vi "FPGA Main.vi"() -> ()   [LabVIEW 2016]
doc: "This example transmits one frame contained in Data Frame every time the Write button is pressed. After building this FPGA VI, you run it using CAN Channel Transmit (Host).vi (not standalone).\n\nThis example assumes the following configuration for CAN 0: Auto Start = True, Listen Only = False, Input Timeout = 10000ms, Output Timeout = 10000ms. The CAN Output node is configured to use an array of U32 for the CAN frame. For more information on configuration, refer to the Help for the NI 9853 CAN module."
uses:
  <vilib>/rvi/eio/common/nirviEmuTemplateMethod_errors.vi
  <vilib>/rvi/Emulation/niFpgaCriticalErrorInLSC.vi
  <vilib>/rvi/eio/common/nirviEmuReportErrorAndStop.vi
  <vilib>/rvi/errors/nirviReportUnexpectedCaseInternalError.vi
  <vilib>/rvi/errors/nirviReportUnexpectedCaseInternalError (U32).vi
  <vilib>/rvi/Emulation/niFpgaProcessEmulError.vi
  <vilib>/rvi/occurrence/nirviWaitOnOccurrenceBase.vi
  <vilib>/rvi/FIFO/Fifo_Resource/nirvififoEmulationReleaseLock.vi
  <vilib>/rvi/FIFO/Fifo_Resource/nirvififoEmulationObtainLock.vi
  <vilib>/rvi/FIFO/Fifo_Resource/nirvififoEmulationCreateLock.vi
  <vilib>/rvi/DataTransferAndStorage/Container/Common/niFpgaContainerGetUniqueNameForEmu.vi
  <vilib>/rvi/FIFO/Fifo_Resource/nirvififoEmulationSetSize.vi
  <vilib>/Utility/error.llb/Clear Errors.vi
  <vilib>/rvi/FIFO/Fifo_Resource/nirviFifoEmulationQueueMgr.vi
  <instcachedir>/0/nirviFifoEmulationQueueMgr_E5CAEC123FF24DC58D834DCA3CDAA9B5.lvgen/nirviFifoEmulationQueueMgr_E5CAEC123FF24DC58D834DCA3CDAA9B5_009.vi
  <vilib>/rvi/errors/niFpgaSetErrorForExecOnDevCompSimple.vi
  <vilib>/rvi/Emulation/niFpgaSctlEmulationGetInTimedLoop.vi
  <vilib>/rvi/Emulation/niFpgaEmulationIsFPGAContextNoSignature.vi
  <vilib>/rvi/Emulation/niFpgaEmulationReportErrorSimple.vi
  <vilib>/rvi/Emulation/niFpgaGetClockAttributes.vi
  <vilib>/rvi/FIFO/Fifo_Resource/nirvififoEmulationDetermineInputValidOut.vi
  <vilib>/eio/EIONode/EIONode.xnode
  <vilib>/rvi/DataTransferAndStorage/Container/XNode/niFpgaContainer.xnode
  <vilib>/rvi/FIFO/Fifo_Resource/nirvififoEmulationRead.vi
  <vilib>/LabVIEW Targets/FPGA/RIO/nicrio_985x_controls.llb/CAN_IO_Frame Array U32.ctl
  <vilib>/rvi/FIFO/Fifo_Resource/nirvififoEmulationWrite.vi
  <vilib>/eio/EIOMethodNode/EIOMethodNode.xnode
  <vilib>/rvi/FIFO/Fifo_Resource/nirvififoEmulationClear.vi
panel:
  out "CAN Frame Out":T1 {"Data" format="%.0x"; "DataLength" format="%.0x"; "InfoB" format="%.0x"; "InfoA" format="%.0x"; "Type" format="%.0x"; "Identifier" format="%.0x"; "Timestamp" format="%.0x"}
  in  "CAN Frame In":T1={"Timestamp"=0, "Identifier"=0, "Type"=0, "InfoA"=0, "InfoB"=0, "DataLength"=0, "Data"=[0, 0, 0, 0, 0, 0, 0, 0]} {"Data" format="%.0x"; "DataLength" format="%.0x"; "InfoB" format="%.0x"; "InfoA" format="%.0x"; "Type" format="%.0x"; "Identifier" format="%.0x"; "Timestamp" format="%.0x"}
  out "FIFO Full":bool
  in  "Write":bool
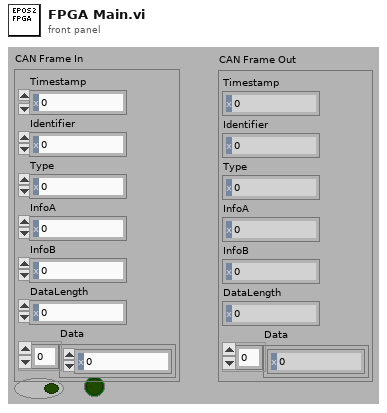
[diagram p1: front panel]
types:
  T1 = cluster{"Timestamp":u64, "Identifier":u32, "Type":u8, "InfoA":u8, "InfoB":u8, "DataLength":u8, "Data":u8[]}
  T2 = typedef "CAN_IO_Frame Array U32.ctl" = u32[]
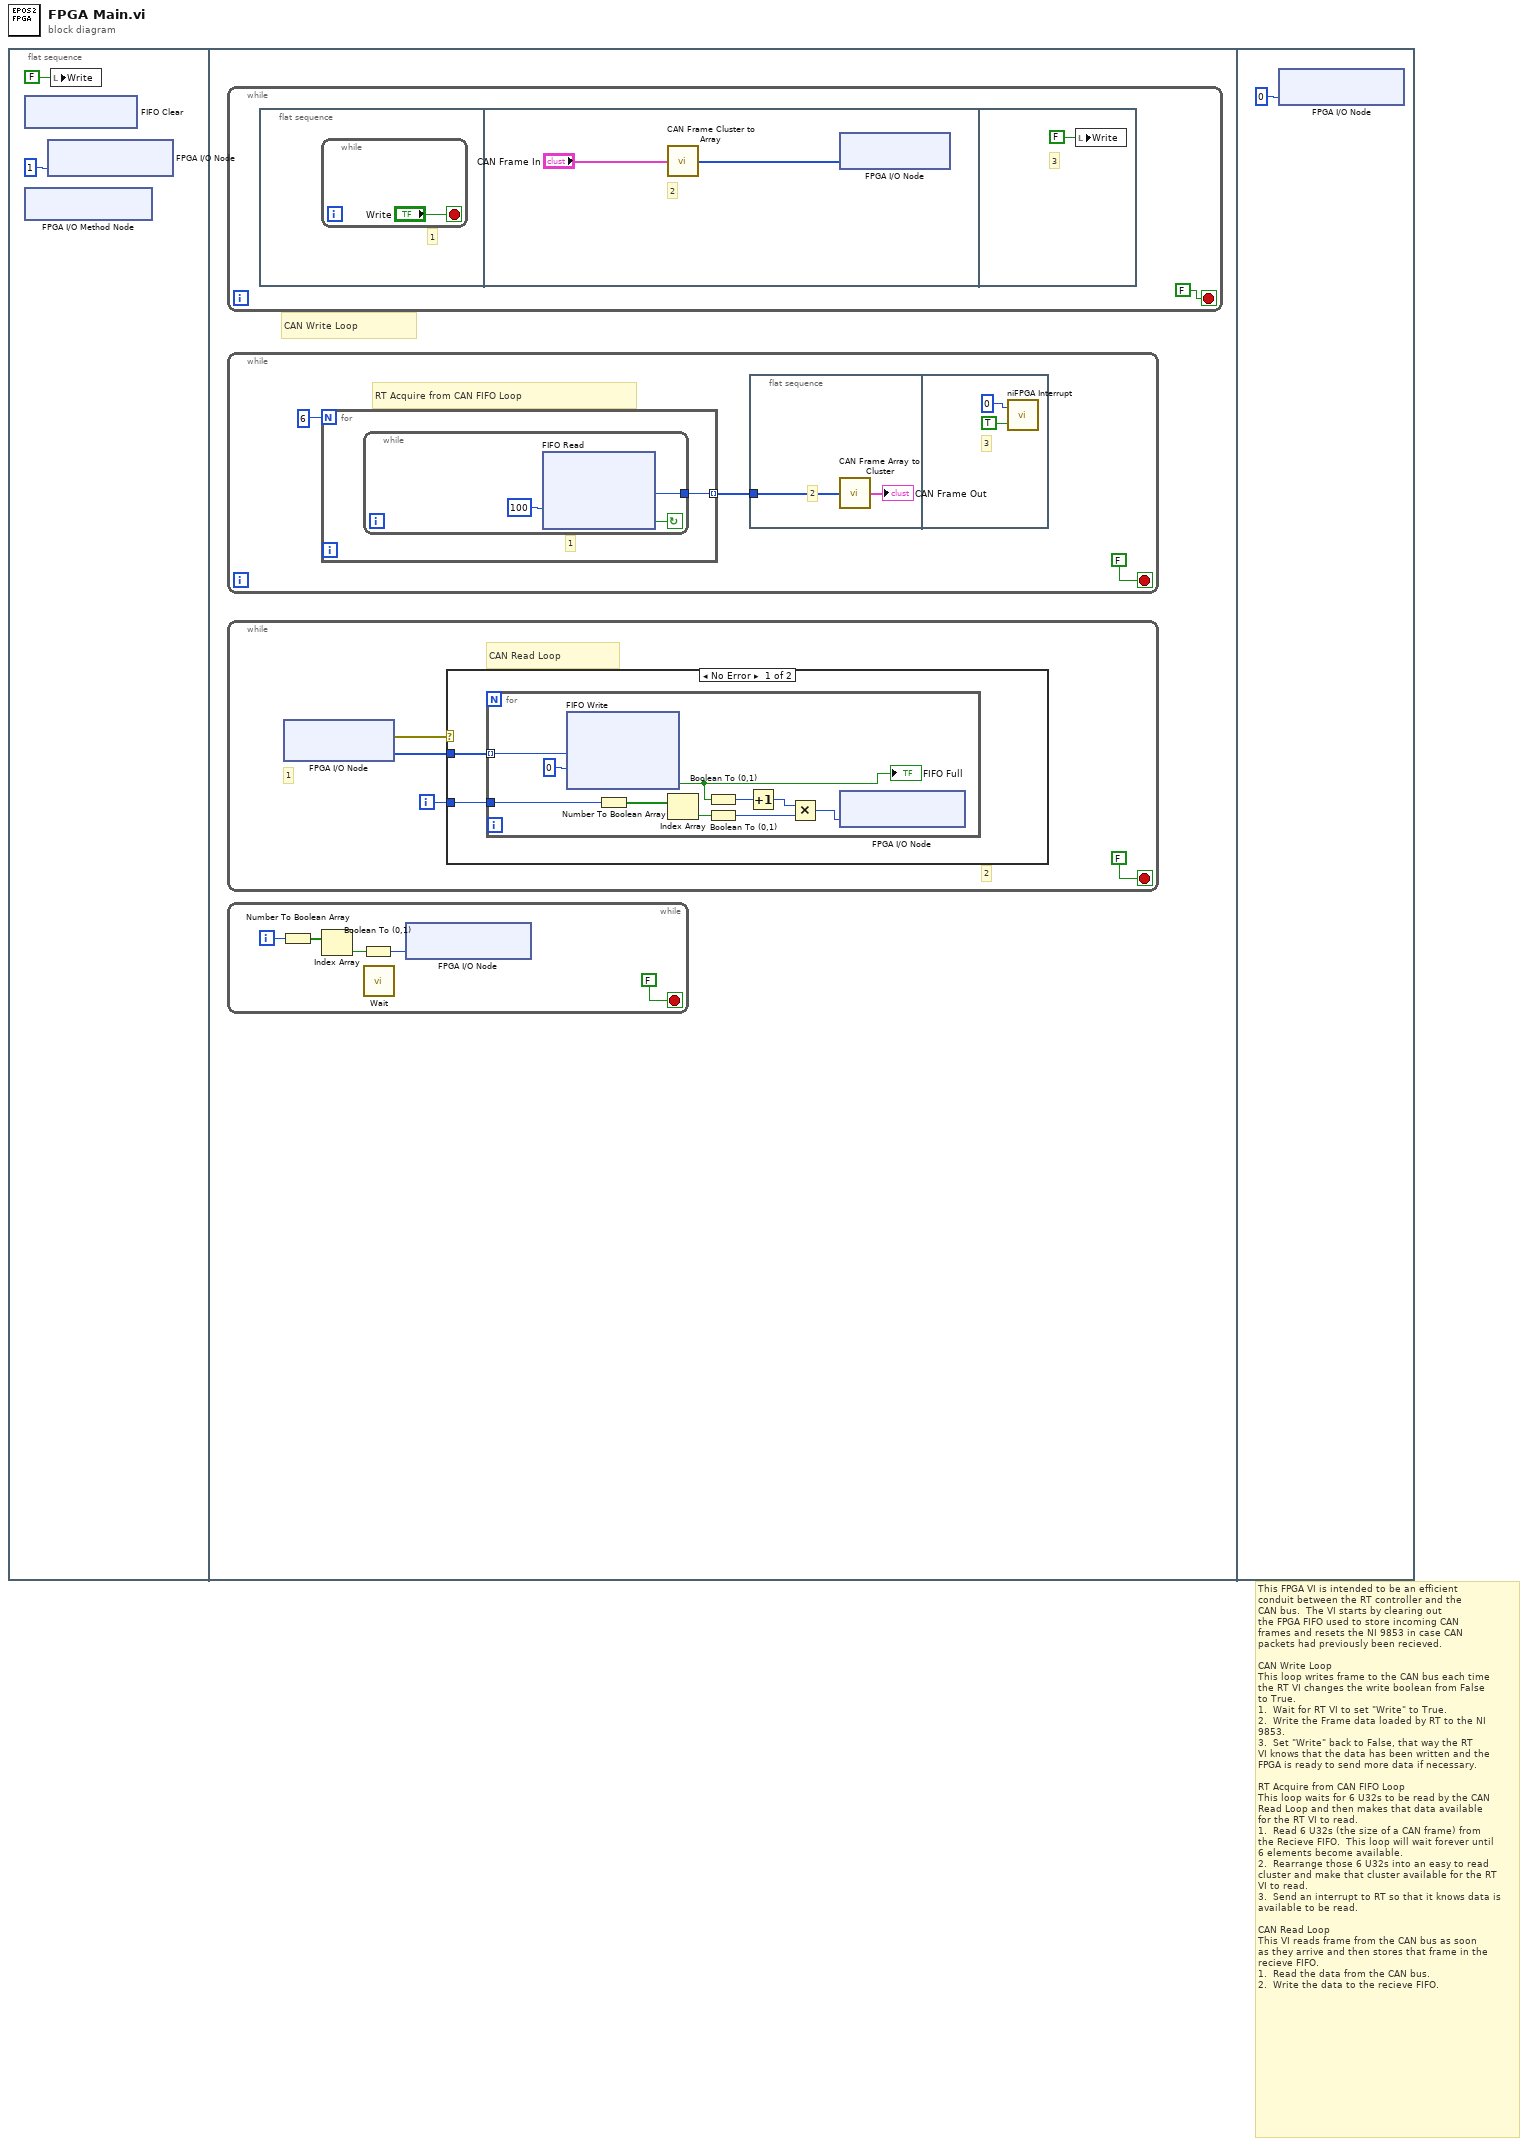
[diagram p0: block diagram]
diagram:
  # "This FPGA VI is intended to be an efficient\nconduit between the RT controller and the\nCAN bus.  The VI starts by clearing out\nthe FPGA FIFO used to store incoming CAN\nframes and resets the NI 9853 in case CAN\npackets had previously been recieved.\n\nCAN Write Loop\nThis loop writes frame to the CAN bus each time\nthe RT VI changes the write boolean from False\nto True.\n1.  Wait for RT VI to set \"Write\" to True.\n2.  Write the Frame data loaded by RT to the NI\n9853.\n3.  Set \"Write\" back to False, that way the RT\nVI knows that the data has been written and the\nFPGA is ready to send more data if necessary.\n\nRT Acquire from CAN FIFO Loop\nThis loop waits for 6 U32s to be read by the CAN\nRead Loop and then makes that data available\nfor the RT VI to read.\n1.  Read 6 U32s (the size of a CAN frame) from\nthe Recieve FIFO.  This loop will wait forever until\n6 elements become available.\n2.  Rearrange those 6 U32s into an easy to read\ncluster and make that cluster available for the RT\nVI to read.\n3.  Send an interrupt to RT so that it knows data is\navailable to be read.\n\nCAN Read Loop\nThis VI reads frame from the CAN bus as soon\nas they arrive and then stores that frame in the\nrecieve FIFO.\n1.  Read the data from the CAN bus.\n2.  Write the data to the recieve FIFO."
  n1 = flat-sequence {
    frame #0 {
      n2 = xnode ("FIFO Clear")() -> ()  [unwired: 1 in, 1 out]
      n3 = xnode "FPGA I/O Method Node"() -> ()  [unwired: 1 in, 1 out]
      n4 = xnode "FPGA I/O Node"("USER FPGA LED"=u8 1) -> ()  [unwired: 1 in, 1 out]
      n5 = local write "Write"(FALSE) -> ()
    }
    frame #1 {
      # "CAN Write Loop"
      n6 = while {
        stop <- FALSE stop-if-true
        n7 = flat-sequence {
          frame #0 {
            # "1"
            n8 = while {
              stop <- "Write" stop-if-true
            }
          }
          frame #1 {
            # "2"
            n9 = call "CAN Frame Cluster to Array.vi"("CAN Frame Cluster In"="CAN Frame In") -> ("CAN Frame Array Out"=w38:u32[])
            n10 = xnode "FPGA I/O Node"("Mod1/CAN1"=w38) -> ()  [unwired: 1 in, 1 out]
          }
          frame #2 {
            # "3"
            n11 = local write "Write"(FALSE ("Write")) -> ()
          }
        }
      }
      n12 = while {
        stop <- FALSE stop-if-true
        # "RT Acquire from CAN FIFO Loop"
        n13 = for {
          N: 6 -> [_]
          tunnel: [w31] -> w24 mode=indexing
          # "1"
          n14 = while {
            tunnel: [w32] -> w31
            stop <- w33 continue-if-true
            n15 = xnode ("FIFO Read")("Timeout"=100 ("Timeout (-1 for no timeout)")) -> ("Element"=w32:u32, "Timed Out?"=w33:bool)  [unwired: 1 in, 1 out]
          }
        }
        n16 = flat-sequence {
          tunnel: w24 -> [w27]
          frame #0 {
            # "2"
            n17 = call "CAN Frame Array to Cluster.vi"("CAN Frame Array In"=w27) -> ("CAN Frame Cluster Out"=→"CAN Frame Out":T1)
          }
          frame #1 {
            # "3"
            n18 = call <vilib>:"niFPGA Interrupt.vi"("Wait Until Cleared (F)"=TRUE ("Wait Until Cleared"), "IRQ Number (0)"=u8 0 ("IRQ Number")) -> ()  [unwired: 1 in]
          }
        }
      }
      n19 = while {
        i -> [w8]
        stop <- FALSE stop-if-true
        # "1"
        # "2"
        # "CAN Read Loop"
        n20 = xnode "FPGA I/O Node"() -> ("error out"=w10:errorcluster, "Mod1/CAN1"=w9:T2)  [unwired: 2 in, 1 out]
        n21 = case shown="No Error" w10 {
          tunnel: w9 -> [w13 _]
          tunnel: w8 -> [w12 _]
          frame No Error {
            n22 = for {
              tunnel: w13 -> [w22] mode=indexing
              tunnel: w12 -> [w14]
              n23 = xnode ("FIFO Write")("Element"=w22, "Timeout"=0) -> ("Timed Out?"=w17:bool)  [unwired: 1 in, 1 out]
              "FIFO Full" <- w17
              n24 = Number To Boolean Array(number=w14) -> (Boolean array=w21:bool[])
              n25 = Index Array(array=w21) -> (element=w18:bool)  [unwired: 1 in]
              n26 = Boolean To (0,1)(Boolean=w17) -> (0, 1=w16:i16)
              n27 = Boolean To (0,1)(Boolean=w18) -> (0, 1=w20:i16)
              n28 = Increment(x=w16) -> (x+1=w15:i16)
              n29 = Multiply(x=w15, y=w20) -> (x*y=w19:i16)
              n30 = xnode "FPGA I/O Node"("USER FPGA LED"=w19) -> ()  [unwired: 1 in, 1 out]
            }
          }
          frame Error {
          }
        }
      }
      n31 = while {
        i -> [w5]
        stop <- FALSE stop-if-true
        n32 = Number To Boolean Array(number=w5) -> (Boolean array=w7:bool[])
        n33 = Index Array(array=w7) -> (element=w6:bool)  [unwired: 1 in]
        n34 = Boolean To (0,1)(Boolean=w6) -> (0, 1=w4:i16)
        n35 = call "Wait"() -> ()  [unwired: 1 in, 1 out]
        n36 = xnode "FPGA I/O Node"("USER FPGA LED"=w4) -> ()  [unwired: 1 in, 1 out]
      }
    }
    frame #2 {
      n37 = xnode "FPGA I/O Node"("USER FPGA LED"=u8 0) -> ()  [unwired: 1 in, 1 out]
    }
  }
